vi "Send Interface Status.vi"(8 "error in (no error)":errorcluster, 10 "Message":string, 11 "Stream in":refnum<class "Stream.lvclass">) -> (0 "error out":errorcluster, 3 "Stream out":refnum<class "Stream.lvclass">)   [LabVIEW 2018, in "Stream.lvclass"]
uses:
  Stream.lvclass
  Interface/Interface.lvclass
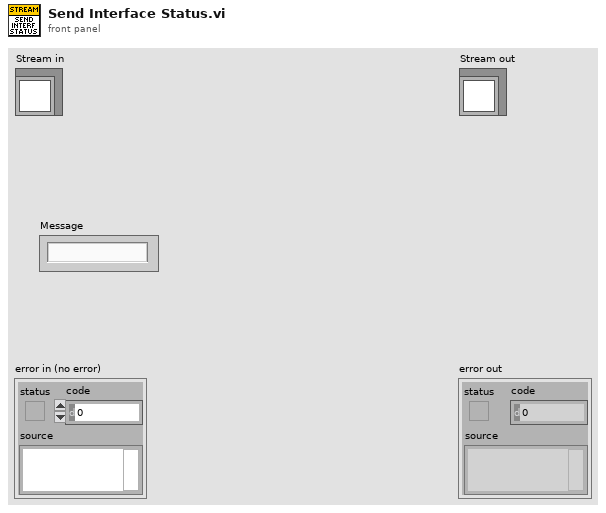
[diagram p1: front panel]
types:
  T1 = cluster{"Current Temperature":i16, "Temperatue Status":string}
  T2 = cluster{"Initialization":bool, "Serial Number":u16}
  T3 = cluster{"EXPTIME":sgl, "PREAMP":u8, "READOUT_RATE":u8, "EM_MODE":u8, "EM_GAIN":u16, "BINNING":u16, "INITIAL_LINE":u16, "INITIAL_COLUMN":u16, "FINAL_LINE":u16, "FINAL_COLUMN":u16, "#FRAMES":u32, "SHUTTER_MODE":u8, "COOLER_POWER_STATUS":u16, "TEMP":i8, "#CUBES":u32, "TRIGGER_MODE":u16}
  T4 = cluster{"CUBE_EXPOSURE_TIME":sgl, "CUBES_DONE":u16, "LAST_IMAGE_NAME":string, "DISK_SPACE":u16, "FRAMES_DONE":u16, "CCD_STATUS":string, "CURRENT_TEMPERATURE":i16, "TEMPERATURE_STATUS":string, "FRAME_EXPOSURE_TIME":u16, "CCD_ON_OFF":bool, "SERIAL_NUMBER":u16, "ACQUIRING":bool}
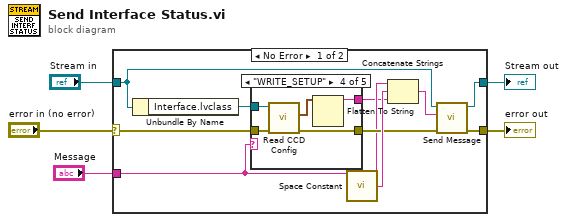
[diagram p0: block diagram]
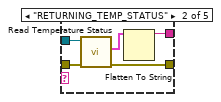
[diagram p3: hidden frame]
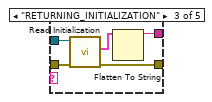
[diagram p4: hidden frame]
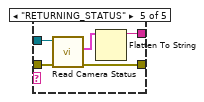
[diagram p5: hidden frame]
diagram:
  n1 = case shown="No Error" "error in (no error)" {
    selector: "error in (no error)" -> [w8 w38]
    tunnel: [w13 w38] -> w4
    tunnel: [w10 w37] -> w2
    tunnel: "Stream in" -> [w11 w37]
    tunnel: "Message" -> [w7 _]
    frame No Error {
      n2 = Unbundle By Name(w11) -> ("Interface.lvclass"=w15:refnum<class "Interface.lvclass">)
      n3 = case shown="\"WRITE_SETUP\"" w7 {
        tunnel: w15 -> [_ w21 w26 w28 w33]
        tunnel: [w16 w20 w25 w29 w34] -> w9
        tunnel: w8 -> [w16 w19 w24 w30 w35]
        tunnel: [_ w17 w22 w31 w36] -> w6
        frame "False", Default {
        }
        frame "RETURNING_TEMP_STATUS" {
          n4 = call "Read Temperature Status.vi"("error in (no error)"=w19, "Interface in"=w21) -> ("error out"=w20:errorcluster, "Temperature Status"=w18:T1)  [unwired: 7 in, 1 out]
          n5 = Flatten To String(anything=w18) -> (data string=w17:string)  [unwired: 3 in, 2 out]
        }
        frame "RETURNING_INITIALIZATION" {
          n6 = call "Read Initialization.vi"("error in (no error)"=w24, "Interface in"=w26) -> ("error out"=w25:errorcluster, "Initialization"=w23:T2)  [unwired: 7 in, 1 out]
          n7 = Flatten To String(anything=w23) -> (data string=w22:string)  [unwired: 3 in, 2 out]
        }
        frame "WRITE_SETUP" {
          n8 = call "Read CCD Config.vi"("error in (no error)"=w30, "Interface in"=w28) -> ("error out"=w29:errorcluster, "CCD Config"=w27:T3)  [unwired: 7 in, 1 out]
          n9 = Flatten To String(anything=w27) -> (data string=w31:string)  [unwired: 3 in, 2 out]
        }
        frame "RETURNING_STATUS" {
          n10 = call "Read Camera Status.vi"("error in (no error)"=w35, "Interface in"=w33) -> ("error out"=w34:errorcluster, "Camera Status"=w32:T4)  [unwired: 7 in, 1 out]
          n11 = Flatten To String(anything=w32) -> (data string=w36:string)  [unwired: 3 in, 2 out]
        }
      }
      n12 = call <vilib>:"Space Constant.vi"() -> ("String"=w14:string)
      n13 = Concatenate Strings(w7, w14, w6) -> (w12:string)
      n14 = call "Send Message.vi"("error in (no error)"=w9, "Message"=w12, "Stream in"=w11) -> ("error out"=w13:errorcluster, "Stream out"=w10:refnum<class "Stream.lvclass">)  [unwired: 7 in]
    }
    frame Error {
    }
  }
  "error out" <- w4
  "Stream out" <- w2
